vi "Setup.vi"(11 "Template Queue in":refnum<class "Template Queue.lvclass">) -> (3 "Template Queue out":refnum<class "Template Queue.lvclass">)   [LabVIEW 2021, in "Template Queue.lvlib" / "Template Queue.lvclass"]
uses:
  Template Queue.lvclass
  Template Queue.lvclass/Template Queue.ctl
  <vilib>/Nathan Davis/jettl/jettl/Queue/Queue.lvclass
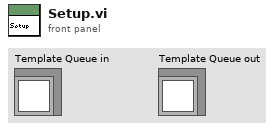
[diagram p1: front panel]
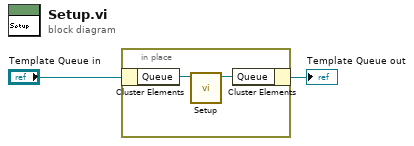
[diagram p0: block diagram]
diagram:
  n1 = in-place {
    n2 = in-place-cluster #1("Template Queue in") -> ("Queue"=w4:refnum<class "Queue.lvclass">)
    n3 = call-dynamic "Setup.vi"("jettl Msg Setup in"=w4) -> ("jettl Msg Setup out"=w3:refnum<class "Queue.lvclass">)  [unwired: 10 in]
    n4 = in-place-cluster #1("Queue"=w3) -> (→"Template Queue out":refnum<class "Template Queue.lvclass">)
  }
